vi "Colormaps and Colorbars.vi"() -> ()   [LabVIEW 2013]
uses:
  <vilib>/Heliosphere Research LLC/Advanced Plotting Toolkit/properties/Colormap.ctl
  <vilib>/Heliosphere Research LLC/Advanced Plotting Toolkit/properties/Colormap_Map.ctl
  <vilib>/Heliosphere Research LLC/Advanced Plotting Toolkit/properties/Colormap_Scaling.ctl
  <vilib>/Heliosphere Research LLC/Advanced Plotting Toolkit/api_plotting/ArrayViewProperties.ctl
  <vilib>/Heliosphere Research LLC/Advanced Plotting Toolkit/properties/Display.ctl
  <vilib>/Heliosphere Research LLC/Advanced Plotting Toolkit/Advanced Plotting Toolkit.lvlib
panel:
  in  "Colormap":T1={"Map"=enum."Automatic", "Value Min"=nan, "Value Max"=nan, "Scaling"=enum."Default", "Reverse"=FALSE}
  out "Color Plot":picture
  # "Colormaps and Colorbars"
  # "Many of the Toolkit VIs use color to visualize data. A\n\"colormap\" determines what color to assign to each data\npoint.\n\nThe colormap settings are determined when the plot is\nmade, through an optional \"Colormap\" entry in the\nproperty cluster.  When a colorbar is later added, its\nappearance is determined automatically from those\nsettings."
  # "Here's the Colormap cluster\nused for this call to ArrayView.vi.\n\n\"Map\" selects which colormap\nto use.  The default is Rainbow.\n\nValue Min and Value Max\ndetermine the range of values\nover which the colormap\napplies.  Try changing them.\n\nLike many other Toolkit\nproperty clusters, \"NaN\" is used\nto specify default behavior; in \nthis case, to use the max and\nmin from the array values."
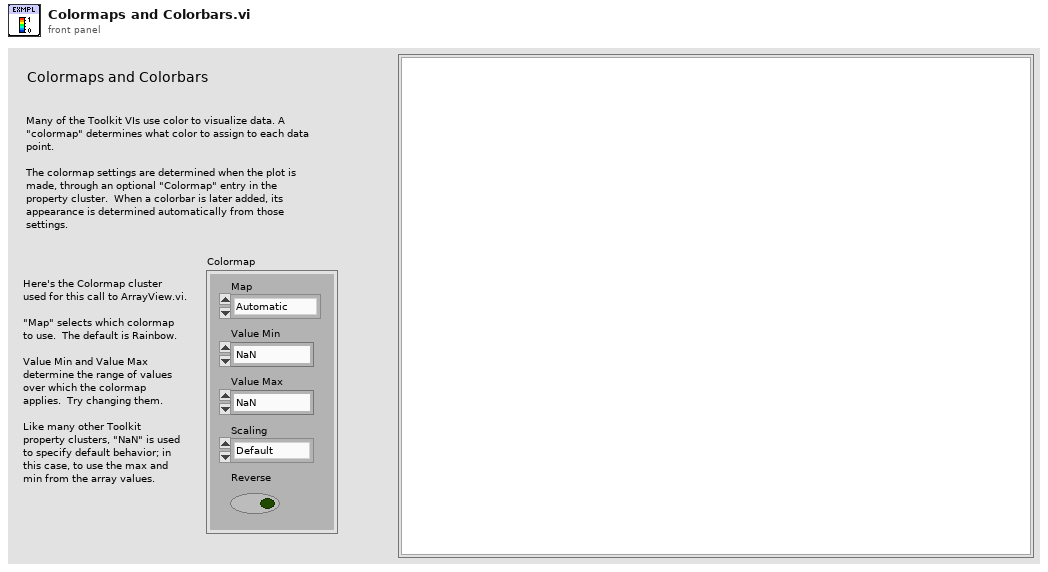
[diagram p1: front panel]
types:
  T1 = typedef "Advanced Plotting Toolkit.lvlib/Colormap.ctl" = cluster{"Map":T2, "Value Min":dbl, "Value Max":dbl, "Scaling":T3, "Reverse":bool}
  T2 = typedef "Advanced Plotting Toolkit.lvlib/Colormap_Map.ctl" = enum16{"Automatic", "Rainbow", "Hot and Cold", "White-Black", "White-Blue", "White-Green", "White-Red", "Fire", "Water", "Earth", "Air", "Pastel", "Banded", "Stepped"}
  T3 = typedef "Advanced Plotting Toolkit.lvlib/Colormap_Scaling.ctl" = enum16{"Default"}
  T4 = typedef "Advanced Plotting Toolkit.lvlib/ArrayViewProperties.ctl" = cluster{"Colormap":T1, "Display":T5}
  T5 = typedef "Advanced Plotting Toolkit.lvlib/Display.ctl" = cluster{"Alpha":dbl, "Z Order":dbl}
  T6 = typedef "Advanced Plotting Toolkit.lvlib/PlotID.ctl" = i32
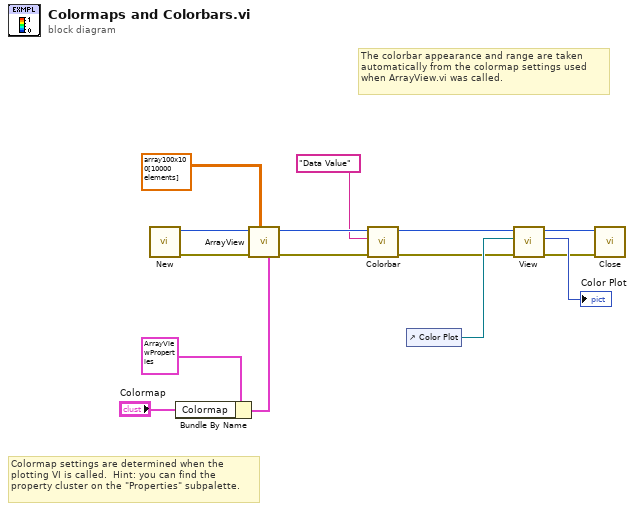
[diagram p0: block diagram]
diagram:
  # "The colorbar appearance and range are taken\nautomatically from the colormap settings used\nwhen ArrayView.vi was called."
  # "Colormap settings are determined when the\nplotting VI is called.  Hint: you can find the\nproperty cluster on the \"Properties\" subpalette."
  n1 = call <vilib>:"New.vi"() -> ("error out"=w11:errorcluster, "Plot ID"=w12:T6)  [unwired: 10 in]
  n2 = Bundle By Name(cluster=T4 {"Colormap"={"Map"=enum."Automatic", "Value Min"=nan, "Value Max"=nan, "Scaling"=enum."Default", "Reverse"=FALSE}, "Display"={"Alpha"=nan, "Z Order"=nan}} ("Array View Properties"), "Colormap"="Colormap") -> (w8:T4)
  n3 = call <vilib>:"ArrayView.vi"("Properties"=w8, "Data"=dbl[][] array100x100[10000 elements] ("x/y"), "error in (no error)"=w11, "Plot ID"=w12) -> ("error out"=w6:errorcluster, "Plot ID Out"=w7:T6)  [unwired: 6 in]
  n4 = call <vilib>:"Colorbar.vi"("error in (no error)"=w6, "Label"="Data Value", "Plot ID"=w7) -> ("error out"=w4:errorcluster, "Plot ID Out"=w5:T6)  [unwired: 7 in]
  n5 = control-ref of="Color Plot"() -> (w15:refnum<vi>)
  n6 = call <vilib>:"View.vi"("error in (no error)"=w4, "Ref for Sizing"=w15, "Plot ID"=w5) -> ("error out"=w1:errorcluster, "Picture"=→"Color Plot":picture, "Plot ID Out"=w13:T6)  [unwired: 6 in]
  n7 = call <vilib>:"Close.vi"("error in (no error)"=w1, "Plot ID"=w13) -> ()  [unwired: 9 in, 1 out]
